vi "GetGlobalDefaultConfiguration_old.vi"(3 "Read defaults?":bool) -> ()   [LabVIEW 2013]
uses:
  QC_MeasurementSetup.vi
panel:
  out "Configuration File Striptest":path
  out "Configuration File Cis":path
  out "Configuration File Stability":path
  out "Configuration File CV":path
  out "Configuration File IV":path
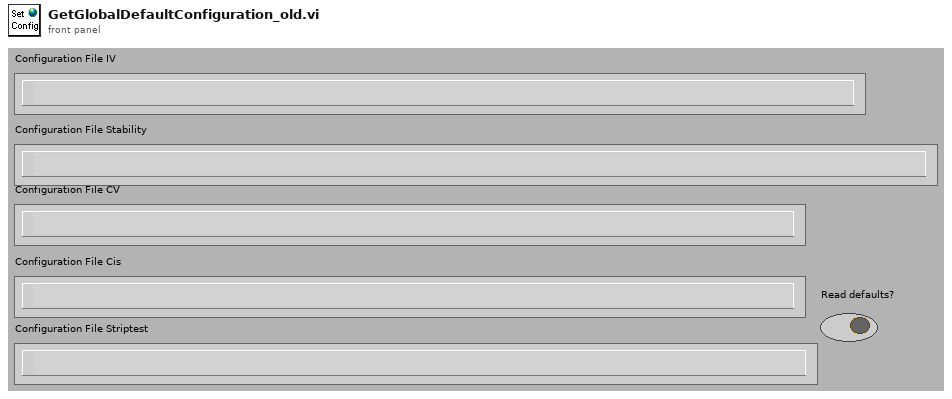
[diagram p1: front panel]
types:
  T1 = cluster{"Supply":refnum<class "SupplyControl.lvclass">, "Arduino":refnum<class "ArduinoControl.lvclass">, "Measurement switch":refnum<class "Switching.lvclass">, "Initial Voltage [V]":dbl, "Final Voltage [V]":dbl, "Step Size [V]":dbl, "Step Interval [s]":i32, "Number Of Steps":u32, "Ramp down steps [V]":dbl, "Ramp down Interval [s]":i32, "hold steps":i32, "Set Current Limit?":bool, "Current Limit [µA]":dbl, "Temperature Readout":enum16{"Read Arduino", "Enter manually"}, "Supply Name":string, "V_breakdown Limit [V]":dbl, "Measurement switch used?":bool}
  T2 = cluster{"Supply":refnum<class "SupplyControl.lvclass">, "LCR":refnum<class "LCRControl.lvclass">, "Arduino":refnum<class "ArduinoControl.lvclass">, "Measurement switch":refnum<class "Switching.lvclass">, "Initial Voltage [V]":dbl, "Final Voltage [V]":dbl, "Step Size [V]":dbl, "Step Interval [s]":i32, "Number Of Steps":u32, "AC frequency [Hz]":i32, "RC Configuration":u16, "AC amplitude [V]":dbl, "Ramp down steps [V]":dbl, "Ramp down Interval [s]":i32, "Set Current Limit?":bool, "Current Limit [µA]":dbl, "Temperature Readout":enum16{"Read Arduino", "Enter manually"}, "Supply Name":string, "LCR Name":string, "V_depletion Limit [V]":dbl, "Measurement switch used?":bool}
  T3 = cluster{"Supply":refnum<class "SupplyControl.lvclass">, "DMM":refnum<class "MultimeterControl.lvclass">, "DUT switch":refnum<class "Switching.lvclass">, "Arduino":refnum<class "ArduinoControl.lvclass">, "Measurement switch":refnum<class "Switching.lvclass">, "Voltage [V]":dbl, "Measurement Interval [s]":i32, "Test Duration":u32, "Ramp up steps [V]":dbl, "Ramp up Interval [s]":u32, "Ramp down steps [V]":dbl, "Ramp down Interval [s]":i32, "Set Current Limit?":bool, "Current Limit [µA]":dbl, "Temperature Readout":enum16{"Read Arduino", "Enter manually"}, "Supply Name":string, "DMM Name":string, "Maximum current fluctuation [%]":dbl, "Measurement switch used?":bool, "DUT switch used?":bool}
  T4 = cluster{"Supply":refnum<class "SupplyControl.lvclass">, "LCR":refnum<class "LCRControl.lvclass">, "Arduino":refnum<class "ArduinoControl.lvclass">, "Measurement switch":refnum<class "Switching.lvclass">, "Initial Voltage [V]":dbl, "Final Voltage [V]":dbl, "Step Size [V]":dbl, "Step Interval [s]":i32, "Number Of Steps":u32, "AC frequency [Hz]":i32, "RC Configuration":u16, "AC amplitude [V]":dbl, "Ramp down steps [V]":dbl, "Ramp down Interval [s]":i32, "Set Current Limit?":bool, "Current Limit [µA]":dbl, "Temperature Readout":enum16{"Read Arduino", "Enter manually"}, "Supply Name":string, "LCR Name":string, "C_is Limit [pF/cm]":dbl, "Measurement switch used?":bool}
  T5 = cluster{"Bias Supply":refnum<class "SupplyControl.lvclass">, "SMU":refnum<class "SupplyControl.lvclass">, "LCR":refnum<class "LCRControl.lvclass">, "ProbeStation":refnum<class "ProbeStationControl.lvclass">, "Arduino":refnum<class "ArduinoControl.lvclass">, "Measurement switch":refnum<class "Switching.lvclass">, "Probe Card Channels":i32, "Bias Voltage [V]":dbl, "First strip":i32, "Last strip":i32, "Base Voltage [V]":dbl, "Base Ramp Step [V]":dbl, "Base Ramp Interval [ms]":u32, "High Voltage [V]":dbl, "High Ramp Step [V]":dbl, "High Ramp Interval [ms]":u32, "AC frequency [Hz]":i32, "AC amplitude [V]":dbl, "RC Configuration":u16, "Single Needle":bool, "Temperature Readout":enum16{"Read Arduino", "Enter manually"}, "Fraction of good strips [%]":dbl, "Measurement switch used?":bool, "Matrix X Channels":cluster{"Mux1 C1":i32, "Mux1 C2":i32, "Mux2 C1":i32, "Mux2 C2":i32}, "Pinholes Y/N":bool, "Capacitance Y/N":bool, "Resistance Y/N":bool, "Bias Supply Name":string, "SMU Name":string, "LCR Name":string}
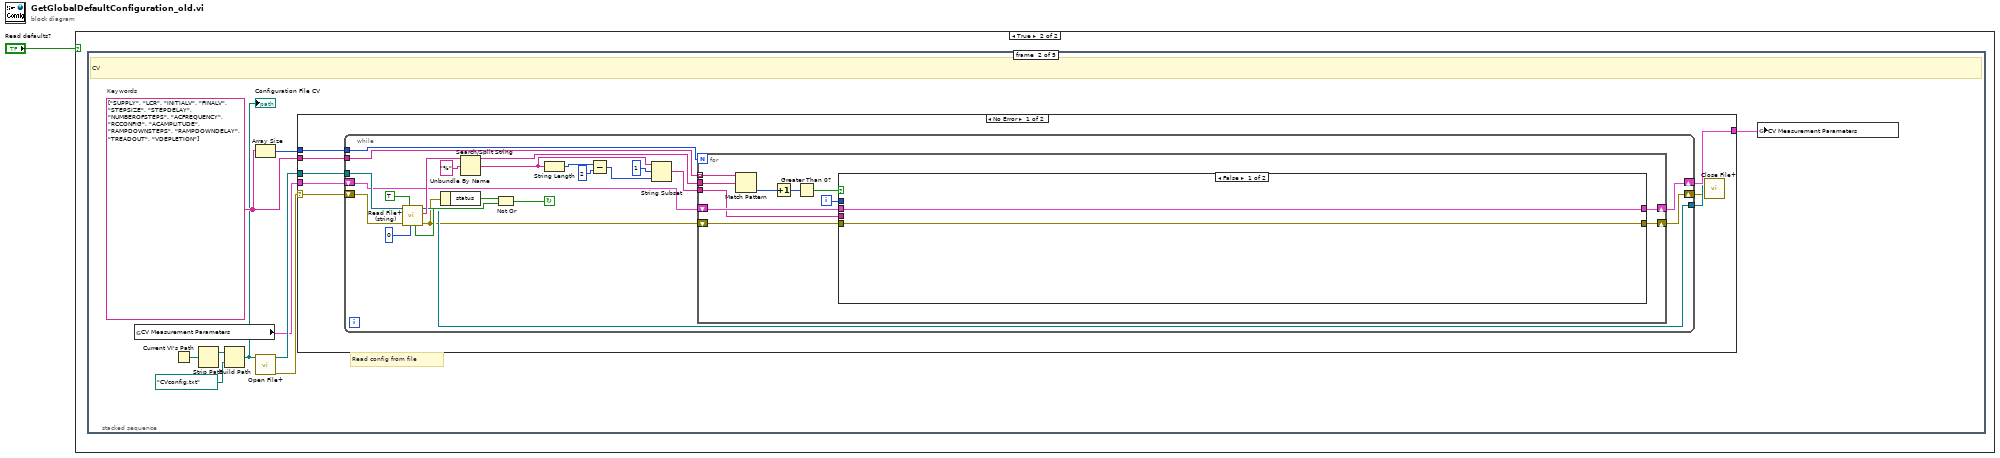
[diagram p0: block diagram]
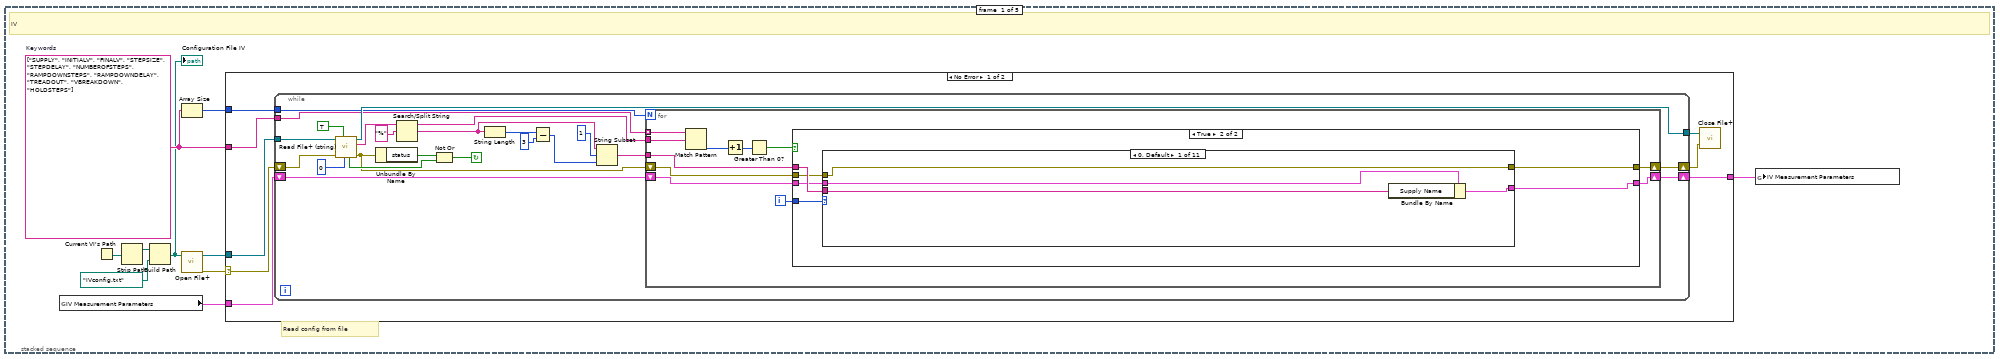
[diagram p3: hidden frame]
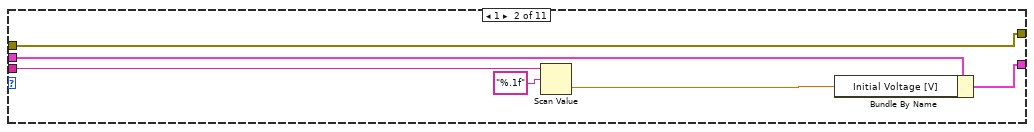
[diagram p5: hidden frame]
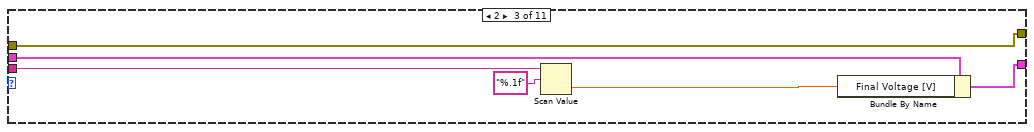
[diagram p6: hidden frame]
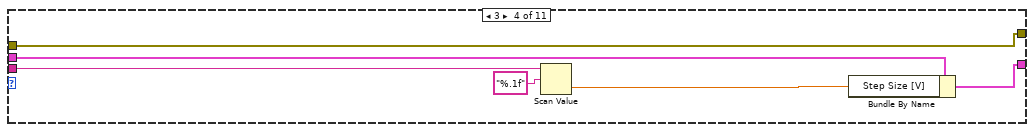
[diagram p7: hidden frame]
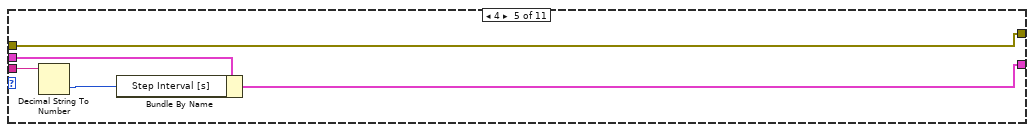
[diagram p8: hidden frame]
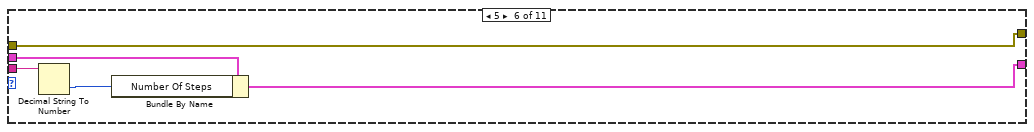
[diagram p9: hidden frame]
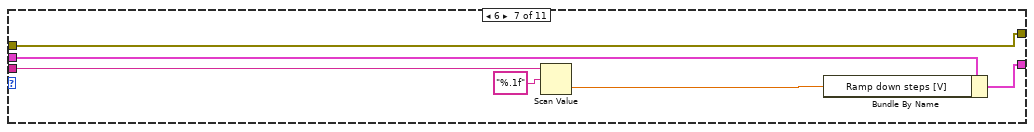
[diagram p10: hidden frame]
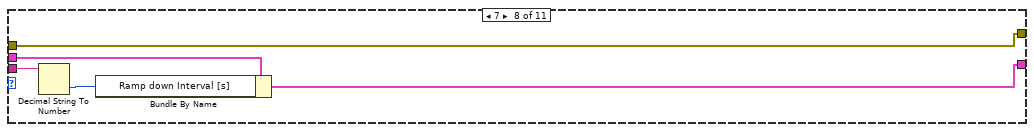
[diagram p11: hidden frame]
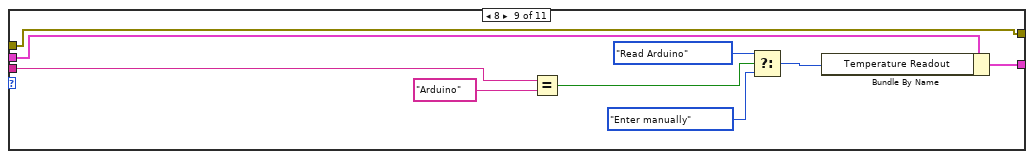
[diagram p12: hidden frame]
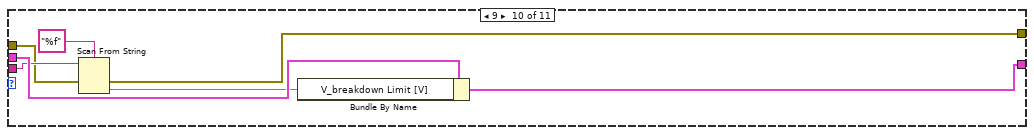
[diagram p13: hidden frame]
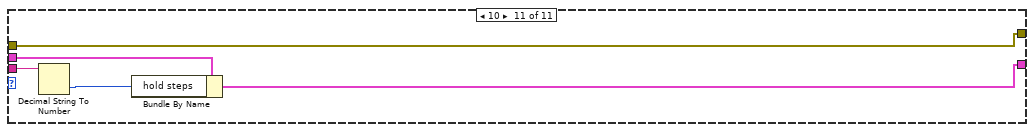
[diagram p14: hidden frame]
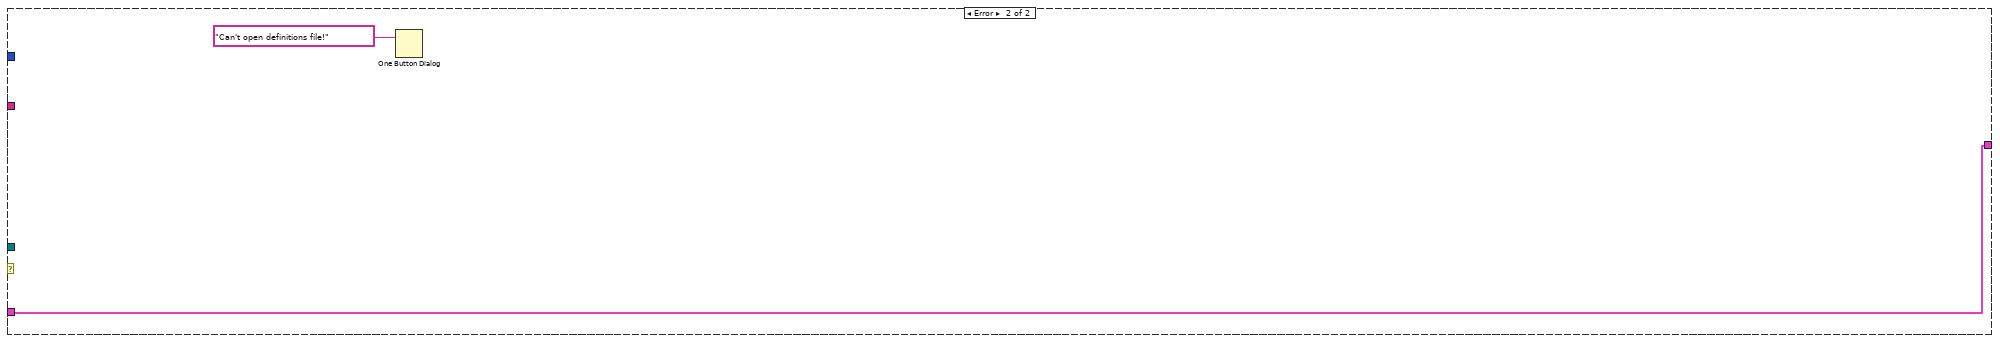
[diagram p15: hidden frame]
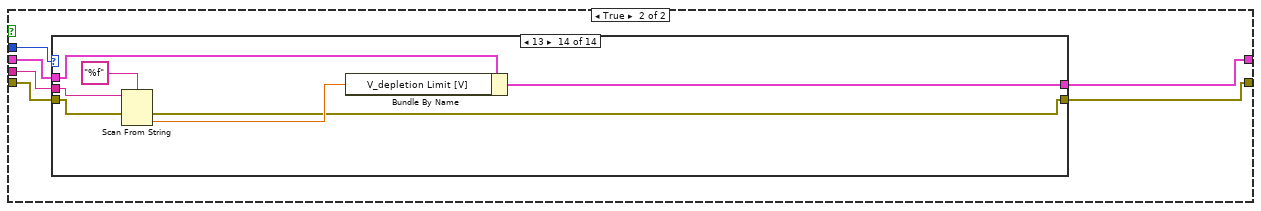
[diagram p16: hidden frame]
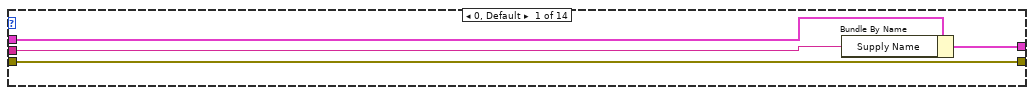
[diagram p17: hidden frame]
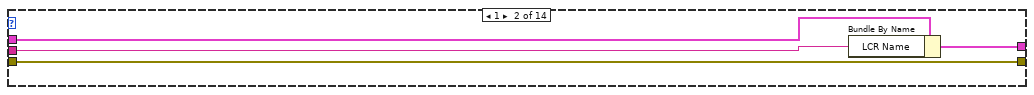
[diagram p18: hidden frame]
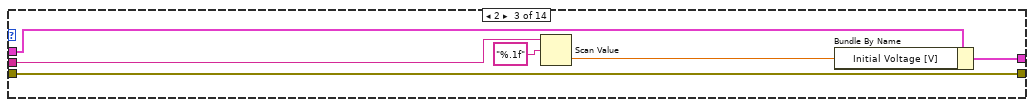
[diagram p19: hidden frame]
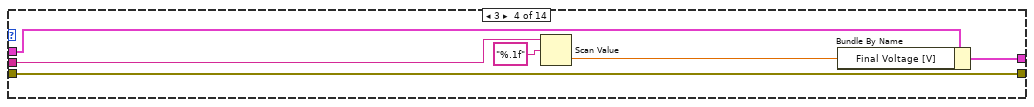
[diagram p20: hidden frame]
diagram:
  n1 = case shown="True" "Read defaults?" {
    frame False {
    }
    frame True {
      n2 = stacked-sequence {
        frame #0 {
          w11 = string[] ["SUPPLY", "INITIALV", "FINALV", "STEPSIZE", "STEPDELAY", "NUMBEROFSTEPS", "RAMPDOWNSTEPS", "RAMPDOWNDELAY", "TREADOUT", "VBREAKDOWN", "HOLDSTEPS"]  # Keywords
          # "Read config from file"
          # "IV"
          n3 = global read "QC_MeasurementSetup.vi" "IV Measurement Parameters"() -> (w2:T1)
          n4 = Current VI's Path() -> (path=w6:path)
          n5 = Strip Path(path=w6) -> (stripped path=w5:path)  [unwired: 1 out]
          n6 = Build Path(base path=w5, name or relative path=path "IVconfig.txt") -> (appended path=w4:path)
          "Configuration File IV" <- w4
          n7 = Array Size(array=w11) -> (size(s)=w10:i32)
          n8 = call <vilib>:"Open File+.vi"("file path (\" \")"=w4) -> ("error out"=w7:errorcluster, "refnum"=w8:refnum<file>)  [unwired: 7 in, 2 out]
          n9 = case shown="No Error" w7 {
            selector: w7 -> [w12 _]
            tunnel: w8 -> [w19 _]
            tunnel: w11 -> [w18 _]
            tunnel: w10 -> [w17 _]
            tunnel: w2 -> [w16 w126]
            tunnel: [w15 w126] -> w3
            frame No Error {
              n10 = while {
                shift-left: w16 -> [w25]
                shift-right: [w23] -> w15
                tunnel: w17 -> [w22]
                tunnel: w18 -> [w28]
                tunnel: [w33] -> w14
                tunnel: w19 -> [w39]
                shift-right: [w20] -> w13
                shift-left: w12 -> [w32]
                stop <- w35 continue-if-true
                n11 = call <vilib>:"Read File+ (string).vi"("count"=0, "line mode (characters:F)"=TRUE, "error in (no error)"=w32, "refnum"=w39) -> ("error out"=w21:errorcluster, "string"=w34:string, "dup refnum"=w33:refnum<file>, "EOF?"=w37:bool)  [unwired: 3 in, 1 out]
                n12 = Unbundle By Name(w21) -> ("status"=w36:bool)
                n13 = Search/Split String(string=w34, search string/char (-)="%" ("search char (-)")) -> (substring before match=w27:string, match + rest of string=w40:string)  [unwired: 1 in, 1 out]
                n14 = Not Or(1:w37, 2:w36) -> (0:w35:bool)
                n15 = String Length(string=w40) -> (length=w26:i32)
                n16 = Subtract(x=w26, y=3) -> (x-y=w29:i32)
                n17 = String Subset(string=w40, offset (0)=1, length (rest)=w29) -> (substring=w24:string)
                n18 = for {
                  N: w22 -> [_]
                  tunnel: w28 -> [w51] mode=indexing
                  tunnel: w27 -> [w46]
                  shift-right: [w47] -> w23
                  shift-left: w25 -> [w48]
                  tunnel: w24 -> [w45]
                  shift-right: [w43] -> w20
                  shift-left: w21 -> [w44]
                  i -> [w49]
                  n19 = Match Pattern(string=w51, regular expression=w46) -> (offset past match=w52:i32)  [unwired: 1 in, 3 out]
                  n20 = Increment(x=w52) -> (x+1=w53:i32)
                  n21 = Greater Than 0?(x=w53) -> (x > 0?=w50:bool)
                  n22 = case shown="True" w50 {
                    tunnel: w49 -> [_ w61]
                    tunnel: w45 -> [_ w60]
                    tunnel: w48 -> [w55 w59]
                    tunnel: [w55 w58] -> w47
                    tunnel: w44 -> [w54 w57]
                    tunnel: [w54 w56] -> w43
                    frame False {
                    }
                    frame True {
                      n23 = case shown="0, Default" w61 {
                        tunnel: w60 -> [w63 w69 w74 w80 w86 w91 w96 w102 w111 w118 w122]
                        tunnel: w59 -> [w64 w71 w77 w83 w88 w93 w99 w104 w113 w120 w125]
                        tunnel: [w65 w70 w76 w82 w87 w92 w98 w103 w112 w119 w124] -> w58
                        tunnel: w57 -> [w62 w66 w72 w78 w84 w89 w94 w100 w110 w115 w121]
                        tunnel: [w62 w66 w72 w78 w84 w89 w94 w100 w110 w114 w121] -> w56
                        frame 0, Default {
                          n24 = Bundle By Name(cluster=w64, "Supply Name"=w63) -> (w65:T1)
                        }
                        frame 1 {
                          n25 = Scan Value(string=w69, format string="%.1f") -> (value=w68:dbl)  [unwired: 1 in, 1 out]
                          n26 = Bundle By Name(cluster=w71, "Initial Voltage [V]"=w68) -> (w70:T1)
                        }
                        frame 2 {
                          n27 = Scan Value(string=w74, format string="%.1f") -> (value=w73:dbl)  [unwired: 1 in, 1 out]
                          n28 = Bundle By Name(cluster=w77, "Final Voltage [V]"=w73) -> (w76:T1)
                        }
                        frame 3 {
                          n29 = Scan Value(string=w80, format string="%.1f") -> (value=w79:dbl)  [unwired: 1 in, 1 out]
                          n30 = Bundle By Name(cluster=w83, "Step Size [V]"=w79) -> (w82:T1)
                        }
                        frame 4 {
                          n31 = Decimal String To Number(string=w86) -> (number=w85:i32)  [unwired: 2 in, 1 out]
                          n32 = Bundle By Name(cluster=w88, "Step Interval [s]"=w85) -> (w87:T1)
                        }
                        frame 5 {
                          n33 = Decimal String To Number(string=w91) -> (number=w90:i32)  [unwired: 2 in, 1 out]
                          n34 = Bundle By Name(cluster=w93, "Number Of Steps"=w90) -> (w92:T1)
                        }
                        frame 6 {
                          n35 = Scan Value(string=w96, format string="%.1f") -> (value=w95:dbl)  [unwired: 1 in, 1 out]
                          n36 = Bundle By Name(cluster=w99, "Ramp down steps [V]"=w95) -> (w98:T1)
                        }
                        frame 7 {
                          n37 = Decimal String To Number(string=w102) -> (number=w101:i32)  [unwired: 2 in, 1 out]
                          n38 = Bundle By Name(cluster=w104, "Ramp down Interval [s]"=w101) -> (w103:T1)
                        }
                        frame 8 {
                          n39 = Equal?(x=w111, y="Arduino") -> (x = y?=w108:bool)
                          n40 = Select(t=enum16{"Read Arduino", "Enter manually"}."Read Arduino" ("Temperature Readout"), s=w108, f=enum16{"Read Arduino", "Enter manually"}."Enter manually" ("Temperature Readout")) -> (s? t:f=w105:enum16{"Read Arduino", "Enter manually"})
                          n41 = Bundle By Name(cluster=w113, "Temperature Readout"=w105) -> (w112:T1)
                        }
                        frame 9 {
                          n42 = Scan From String(format string="%f", input string=w118, error in=w115) -> (error out=w114:errorcluster, output 1=w117:dbl)  [unwired: 2 in, 2 out]
                          n43 = Bundle By Name(cluster=w120, "V_breakdown Limit [V]"=w117) -> (w119:T1)
                        }
                        frame 10 {
                          n44 = Decimal String To Number(string=w122) -> (number=w123:i32)  [unwired: 2 in, 1 out]
                          n45 = Bundle By Name(cluster=w125, "hold steps"=w123) -> (w124:T1)
                        }
                      }
                    }
                  }
                }
              }
              n46 = call <vilib>:"Close File+.vi"("error in (no error)"=w13, "refnum"=w14) -> ()  [unwired: 3 in, 3 out]
            }
            frame Error {
              n47 = One Button Dialog(message="Can't open definitions file!") -> ()  [unwired: 1 in, 1 out]
            }
          }
          n48 = global write "QC_MeasurementSetup.vi" "IV Measurement Parameters"(w3) -> ()
        }
        frame #1 {
          w137 = string[] ["SUPPLY", "LCR", "INITIALV", "FINALV", "STEPSIZE", "STEPDELAY", "NUMBEROFSTEPS", "ACFREQUENCY", "RCCONFIG", "ACAMPLITUDE", "RAMPDOWNSTEPS", "RAMPDOWNDELAY", "TREADOUT", "VDEPLETION"]  # Keywords
          # "Read config from file"
          # "CV"
          n49 = global read "QC_MeasurementSetup.vi" "CV Measurement Parameters"() -> (w128:T2)
          n50 = Current VI's Path() -> (path=w132:path)
          n51 = Strip Path(path=w132) -> (stripped path=w131:path)  [unwired: 1 out]
          n52 = Build Path(base path=w131, name or relative path=path "CVconfig.txt") -> (appended path=w130:path)
          "Configuration File CV" <- w130
          n53 = Array Size(array=w137) -> (size(s)=w136:i32)
          n54 = call <vilib>:"Open File+.vi"("file path (\" \")"=w130) -> ("error out"=w133:errorcluster, "refnum"=w134:refnum<file>)  [unwired: 7 in, 2 out]
          n55 = case shown="No Error" w133 {
            selector: w133 -> [w138 _]
            tunnel: w134 -> [w145 _]
            tunnel: w137 -> [w144 _]
            tunnel: w136 -> [w143 _]
            tunnel: w128 -> [w142 w271]
            tunnel: [w141 w271] -> w129
            frame No Error {
              n56 = while {
                shift-left: w142 -> [w151]
                shift-right: [w149] -> w141
                tunnel: w143 -> [w148]
                tunnel: w144 -> [w154]
                tunnel: [w159] -> w140
                tunnel: w145 -> [w165]
                shift-right: [w146] -> w139
                shift-left: w138 -> [w158]
                stop <- w161 continue-if-true
                n57 = call <vilib>:"Read File+ (string).vi"("count"=0, "line mode (characters:F)"=TRUE, "error in (no error)"=w158, "refnum"=w165) -> ("error out"=w147:errorcluster, "string"=w160:string, "dup refnum"=w159:refnum<file>, "EOF?"=w163:bool)  [unwired: 3 in, 1 out]
                n58 = Unbundle By Name(w147) -> ("status"=w162:bool)
                n59 = Search/Split String(string=w160, search string/char (-)="%" ("search char (-)")) -> (substring before match=w153:string, match + rest of string=w166:string)  [unwired: 1 in, 1 out]
                n60 = Not Or(1:w163, 2:w162) -> (0:w161:bool)
                n61 = String Length(string=w166) -> (length=w152:i32)
                n62 = Subtract(x=w152, y=2) -> (x-y=w155:i32)
                n63 = String Subset(string=w166, offset (0)=1, length (rest)=w155) -> (substring=w150:string)
                n64 = for {
                  N: w148 -> [_]
                  tunnel: w154 -> [w177] mode=indexing
                  tunnel: w153 -> [w172]
                  shift-right: [w173] -> w149
                  shift-left: w151 -> [w174]
                  tunnel: w150 -> [w171]
                  shift-right: [w169] -> w146
                  shift-left: w147 -> [w170]
                  i -> [w175]
                  n65 = Match Pattern(string=w177, regular expression=w172) -> (offset past match=w178:i32)  [unwired: 1 in, 3 out]
                  n66 = Increment(x=w178) -> (x+1=w179:i32)
                  n67 = Greater Than 0?(x=w179) -> (x > 0?=w176:bool)
                  n68 = case shown="False" w176 {
                    tunnel: w175 -> [_ w187]
                    tunnel: w171 -> [_ w186]
                    tunnel: w174 -> [w181 w185]
                    tunnel: [w181 w184] -> w173
                    tunnel: w170 -> [w180 w183]
                    tunnel: [w180 w182] -> w169
                    frame False {
                    }
                    frame True {
                      n69 = case shown="13" w187 {
                        tunnel: w186 -> [w189 w193 w199 w204 w210 w216 w221 w226 w234 w243 w246 w252 w261 w268]
                        tunnel: w185 -> [w190 w194 w201 w207 w213 w218 w223 w228 w237 w241 w249 w254 w263 w264]
                        tunnel: [w191 w195 w200 w206 w212 w217 w222 w227 w236 w239 w248 w253 w262 w265] -> w184
                        tunnel: w183 -> [w188 w192 w196 w202 w208 w214 w219 w224 w229 w238 w244 w250 w260 w267]
                        tunnel: [w188 w192 w196 w202 w208 w214 w219 w224 w229 w238 w244 w250 w260 w266] -> w182
                        frame 0, Default {
                          n70 = Bundle By Name(cluster=w190, "Supply Name"=w189) -> (w191:T2)
                        }
                        frame 1 {
                          n71 = Bundle By Name(cluster=w194, "LCR Name"=w193) -> (w195:T2)
                        }
                        frame 2 {
                          n72 = Scan Value(string=w199, format string="%.1f") -> (value=w198:dbl)  [unwired: 1 in, 1 out]
                          n73 = Bundle By Name(cluster=w201, "Initial Voltage [V]"=w198) -> (w200:T2)
                        }
                        frame 3 {
                          n74 = Scan Value(string=w204, format string="%.1f") -> (value=w203:dbl)  [unwired: 1 in, 1 out]
                          n75 = Bundle By Name(cluster=w207, "Final Voltage [V]"=w203) -> (w206:T2)
                        }
                        frame 4 {
                          n76 = Scan Value(string=w210, format string="%.1f") -> (value=w209:dbl)  [unwired: 1 in, 1 out]
                          n77 = Bundle By Name(cluster=w213, "Step Size [V]"=w209) -> (w212:T2)
                        }
                        frame 5 {
                          n78 = Decimal String To Number(string=w216) -> (number=w215:i32)  [unwired: 2 in, 1 out]
                          n79 = Bundle By Name(cluster=w218, "Step Interval [s]"=w215) -> (w217:T2)
                        }
                        frame 6 {
                          n80 = Decimal String To Number(string=w221) -> (number=w220:i32)  [unwired: 2 in, 1 out]
                          n81 = Bundle By Name(cluster=w223, "Number Of Steps"=w220) -> (w222:T2)
                        }
                        frame 7 {
                          n82 = Decimal String To Number(string=w226) -> (number=w225:i32)  [unwired: 2 in, 1 out]
                          n83 = Bundle By Name(cluster=w228, "AC frequency [Hz]"=w225) -> (w227:T2)
                        }
                        frame 8 {
                          w233 = u16 0 items=["serial", "parallel"] ("RC Configuration")
                          w232 = u16 1 items=["serial", "parallel"] ("RC Configuration")
                          n84 = Equal?(x=w234, y="serial") -> (x = y?=w231:bool)
                          n85 = Select(t=w233, s=w231, f=w232) -> (s? t:f=w230:u16)
                          n86 = Bundle By Name(cluster=w237, "RC Configuration"=w230) -> (w236:T2)
                        }
                        frame 9 {
                          n87 = Scan Value(string=w243, format string="%.1f") -> (value=w240:dbl)  [unwired: 1 in, 1 out]
                          n88 = Bundle By Name(cluster=w241, "AC amplitude [V]"=w240) -> (w239:T2)
                        }
                        frame 10 {
                          n89 = Scan Value(string=w246, format string="%.1f") -> (value=w245:dbl)  [unwired: 1 in, 1 out]
                          n90 = Bundle By Name(cluster=w249, "Ramp down steps [V]"=w245) -> (w248:T2)
                        }
                        frame 11 {
                          n91 = Decimal String To Number(string=w252) -> (number=w251:i32)  [unwired: 2 in, 1 out]
                          n92 = Bundle By Name(cluster=w254, "Ramp down Interval [s]"=w251) -> (w253:T2)
                        }
                        frame 12 {
                          n93 = Equal?(x=w261, y="Arduino") -> (x = y?=w258:bool)
                          n94 = Select(t=enum16{"Read Arduino", "Enter manually"}."Read Arduino" ("Temperature Readout"), s=w258, f=enum16{"Read Arduino", "Enter manually"}."Enter manually" ("Temperature Readout")) -> (s? t:f=w255:enum16{"Read Arduino", "Enter manually"})
                          n95 = Bundle By Name(cluster=w263, "Temperature Readout"=w255) -> (w262:T2)
                        }
                        frame 13 {
                          n96 = Scan From String(format string="%f", input string=w268, error in=w267) -> (error out=w266:errorcluster, output 1=w270:dbl)  [unwired: 2 in, 2 out]
                          n97 = Bundle By Name(cluster=w264, "V_depletion Limit [V]"=w270) -> (w265:T2)
                        }
                      }
                    }
                  }
                }
              }
              n98 = call <vilib>:"Close File+.vi"("error in (no error)"=w139, "refnum"=w140) -> ()  [unwired: 3 in, 3 out]
            }
            frame Error {
              n99 = One Button Dialog(message="Can't open definitions file!") -> ()  [unwired: 1 in, 1 out]
            }
          }
          n100 = global write "QC_MeasurementSetup.vi" "CV Measurement Parameters"(w129) -> ()
        }
        frame #2 {
          w282 = string[] ["SUPPLY", "VOLTAGE", "INTERVAL", "DURATION", "RAMPUPSTEPS", "RAMPUPDELAY", "RAMPDOWNSTEPS", "RAMPDOWNDELAY", "TREADOUT", "IFLUCTUATIONS"]  # Keywords
          # "Read config from file"
          # "STABILITY"
          n101 = global read "QC_MeasurementSetup.vi" "Current Stability Measurement Parameters"() -> (w273:T3)
          n102 = Current VI's Path() -> (path=w277:path)
          n103 = Strip Path(path=w277) -> (stripped path=w276:path)  [unwired: 1 out]
          n104 = Build Path(base path=w276, name or relative path=path "STABILITYconfig.txt") -> (appended path=w275:path)
          "Configuration File Stability" <- w275
          n105 = Array Size(array=w282) -> (size(s)=w281:i32)
          n106 = call <vilib>:"Open File+.vi"("file path (\" \")"=w275) -> ("error out"=w278:errorcluster, "refnum"=w279:refnum<file>)  [unwired: 7 in, 2 out]
          n107 = case shown="No Error" w278 {
            selector: w278 -> [w283 _]
            tunnel: w279 -> [w290 _]
            tunnel: w282 -> [w289 _]
            tunnel: w281 -> [w288 _]
            tunnel: w273 -> [w287 w391]
            tunnel: [w286 w391] -> w274
            frame No Error {
              n108 = while {
                shift-left: w287 -> [w296]
                shift-right: [w294] -> w286
                tunnel: w288 -> [w293]
                tunnel: w289 -> [w299]
                tunnel: [w304] -> w285
                tunnel: w290 -> [w310]
                shift-right: [w291] -> w284
                shift-left: w283 -> [w303]
                stop <- w306 continue-if-true
                n109 = call <vilib>:"Read File+ (string).vi"("count"=0, "line mode (characters:F)"=TRUE, "error in (no error)"=w303, "refnum"=w310) -> ("error out"=w292:errorcluster, "string"=w305:string, "dup refnum"=w304:refnum<file>, "EOF?"=w308:bool)  [unwired: 3 in, 1 out]
                n110 = Unbundle By Name(w292) -> ("status"=w307:bool)
                n111 = Search/Split String(string=w305, search string/char (-)="%" ("search char (-)")) -> (substring before match=w298:string, match + rest of string=w311:string)  [unwired: 1 in, 1 out]
                n112 = Not Or(1:w308, 2:w307) -> (0:w306:bool)
                n113 = String Length(string=w311) -> (length=w297:i32)
                n114 = Subtract(x=w297, y=3) -> (x-y=w300:i32)
                n115 = String Subset(string=w311, offset (0)=1, length (rest)=w300) -> (substring=w295:string)
                n116 = for {
                  N: w293 -> [_]
                  tunnel: w299 -> [w322] mode=indexing
                  tunnel: w298 -> [w317]
                  shift-right: [w318] -> w294
                  shift-left: w296 -> [w319]
                  tunnel: w295 -> [w316]
                  shift-right: [w314] -> w291
                  shift-left: w292 -> [w315]
                  i -> [w320]
                  n117 = Match Pattern(string=w322, regular expression=w317) -> (offset past match=w323:i32)  [unwired: 1 in, 3 out]
                  n118 = Increment(x=w323) -> (x+1=w324:i32)
                  n119 = Greater Than 0?(x=w324) -> (x > 0?=w321:bool)
                  n120 = case shown="True" w321 {
                    tunnel: w320 -> [_ w332]
                    tunnel: w316 -> [_ w331]
                    tunnel: w319 -> [w326 w330]
                    tunnel: [w326 w329] -> w318
                    tunnel: w315 -> [w325 w328]
                    tunnel: [w325 w327] -> w314
                    frame False {
                    }
                    frame True {
                      n121 = case shown="7" w332 {
                        tunnel: w331 -> [w333 w340 w344 w349 w355 w361 w366 w372 w381 w387]
                        tunnel: w330 -> [w335 w342 w347 w352 w358 w363 w369 w374 w383 w388]
                        tunnel: [w336 w341 w346 w351 w357 w362 w368 w373 w382 w386] -> w329
                        tunnel: w328 -> [w334 w337 w345 w350 w356 w359 w364 w370 w380 w384]
                        tunnel: [w334 w337 w345 w350 w356 w359 w364 w370 w380 w385] -> w327
                        frame 0, Default {
                          n122 = Bundle By Name(cluster=w335, "Supply Name"=w333) -> (w336:T3)
                        }
                        frame 1 {
                          n123 = Scan Value(string=w340, format string="%.1f") -> (value=w339:dbl)  [unwired: 1 in, 1 out]
                          n124 = Bundle By Name(cluster=w342, "Voltage [V]"=w339) -> (w341:T3)
                        }
                        frame 2 {
                          n125 = Decimal String To Number(string=w344) -> (number=w343:i32)  [unwired: 2 in, 1 out]
                          n126 = Bundle By Name(cluster=w347, "Measurement Interval [s]"=w343) -> (w346:T3)
                        }
                        frame 3 {
                          n127 = Decimal String To Number(string=w349) -> (number=w348:i32)  [unwired: 2 in, 1 out]
                          n128 = Bundle By Name(cluster=w352, "Test Duration"=w348) -> (w351:T3)
                        }
                        frame 4 {
                          n129 = Scan Value(string=w355, format string="%.1f") -> (value=w353:dbl)  [unwired: 1 in, 1 out]
                          n130 = Bundle By Name(cluster=w358, "Ramp up steps [V]"=w353) -> (w357:T3)
                        }
                        frame 5 {
                          n131 = Decimal String To Number(string=w361) -> (number=w360:i32)  [unwired: 2 in, 1 out]
                          n132 = Bundle By Name(cluster=w363, "Ramp up Interval [s]"=w360) -> (w362:T3)
                        }
                        frame 6 {
                          n133 = Scan Value(string=w366, format string="%.1f") -> (value=w365:dbl)  [unwired: 1 in, 1 out]
                          n134 = Bundle By Name(cluster=w369, "Ramp down steps [V]"=w365) -> (w368:T3)
                        }
                        frame 7 {
                          n135 = Decimal String To Number(string=w372) -> (number=w371:i32)  [unwired: 2 in, 1 out]
                          n136 = Bundle By Name(cluster=w374, "Ramp down Interval [s]"=w371) -> (w373:T3)
                        }
                        frame 8 {
                          n137 = Equal?(x=w381, y="Arduino") -> (x = y?=w378:bool)
                          n138 = Select(t=enum16{"Read Arduino", "Enter manually"}."Read Arduino" ("Temperature Readout"), s=w378, f=enum16{"Read Arduino", "Enter manually"}."Enter manually" ("Temperature Readout")) -> (s? t:f=w375:enum16{"Read Arduino", "Enter manually"})
                          n139 = Bundle By Name(cluster=w383, "Temperature Readout"=w375) -> (w382:T3)
                        }
                        frame 9 {
                          n140 = Scan From String(format string="%f", input string=w387, error in=w384) -> (error out=w385:errorcluster, output 1=w390:dbl)  [unwired: 2 in, 2 out]
                          n141 = Bundle By Name(cluster=w388, "Maximum current fluctuation [%]"=w390) -> (w386:T3)
                        }
                      }
                    }
                  }
                }
              }
              n142 = call <vilib>:"Close File+.vi"("error in (no error)"=w284, "refnum"=w285) -> ()  [unwired: 3 in, 3 out]
            }
            frame Error {
              n143 = One Button Dialog(message="Can't open definitions file!") -> ()  [unwired: 1 in, 1 out]
            }
          }
          n144 = global write "QC_MeasurementSetup.vi" "Current Stability Measurement Parameters"(w274) -> ()
        }
        frame #3 {
          w402 = string[] ["SUPPLY", "LCR", "INITIALV", "FINALV", "STEPSIZE", "STEPDELAY", "NUMBEROFSTEPS", "ACFREQUENCY", "RCCONFIG", "ACAMPLITUDE", "RAMPDOWNSTEPS", "RAMPDOWNDELAY", "TREADOUT", "CISLIMIT"]  # Keywords
          # "Read config from file"
          # "CIS"
          n145 = global read "QC_MeasurementSetup.vi" "Cis Measurement Parameters"() -> (w393:T4)
          n146 = Current VI's Path() -> (path=w397:path)
          n147 = Strip Path(path=w397) -> (stripped path=w396:path)  [unwired: 1 out]
          n148 = Build Path(base path=w396, name or relative path=path "CISconfig.txt") -> (appended path=w395:path)
          "Configuration File Cis" <- w395
          n149 = Array Size(array=w402) -> (size(s)=w401:i32)
          n150 = call <vilib>:"Open File+.vi"("file path (\" \")"=w395) -> ("error out"=w398:errorcluster, "refnum"=w399:refnum<file>)  [unwired: 7 in, 2 out]
          n151 = case shown="No Error" w398 {
            selector: w398 -> [w403 _]
            tunnel: w399 -> [w410 _]
            tunnel: w402 -> [w409 _]
            tunnel: w401 -> [w408 _]
            tunnel: w393 -> [w407 w536]
            tunnel: [w406 w536] -> w394
            frame No Error {
              n152 = while {
                shift-left: w407 -> [w416]
                shift-right: [w414] -> w406
                tunnel: w408 -> [w413]
                tunnel: w409 -> [w419]
                tunnel: [w424] -> w405
                tunnel: w410 -> [w430]
                shift-right: [w411] -> w404
                shift-left: w403 -> [w423]
                stop <- w426 continue-if-true
                n153 = call <vilib>:"Read File+ (string).vi"("count"=0, "line mode (characters:F)"=TRUE, "error in (no error)"=w423, "refnum"=w430) -> ("error out"=w412:errorcluster, "string"=w425:string, "dup refnum"=w424:refnum<file>, "EOF?"=w428:bool)  [unwired: 3 in, 1 out]
                n154 = Unbundle By Name(w412) -> ("status"=w427:bool)
                n155 = Search/Split String(string=w425, search string/char (-)="%" ("search char (-)")) -> (substring before match=w418:string, match + rest of string=w431:string)  [unwired: 1 in, 1 out]
                n156 = Not Or(1:w428, 2:w427) -> (0:w426:bool)
                n157 = String Length(string=w431) -> (length=w417:i32)
                n158 = Subtract(x=w417, y=3) -> (x-y=w420:i32)
                n159 = String Subset(string=w431, offset (0)=1, length (rest)=w420) -> (substring=w415:string)
                n160 = for {
                  N: w413 -> [_]
                  tunnel: w419 -> [w442] mode=indexing
                  tunnel: w418 -> [w437]
                  shift-right: [w438] -> w414
                  shift-left: w416 -> [w439]
                  tunnel: w415 -> [w436]
                  shift-right: [w434] -> w411
                  shift-left: w412 -> [w435]
                  i -> [w440]
                  n161 = Match Pattern(string=w442, regular expression=w437) -> (offset past match=w443:i32)  [unwired: 1 in, 3 out]
                  n162 = Increment(x=w443) -> (x+1=w444:i32)
                  n163 = Greater Than 0?(x=w444) -> (x > 0?=w441:bool)
                  n164 = case shown="True" w441 {
                    tunnel: w440 -> [_ w452]
                    tunnel: w436 -> [_ w451]
                    tunnel: w439 -> [w446 w450]
                    tunnel: [w446 w449] -> w438
                    tunnel: w435 -> [w445 w448]
                    tunnel: [w445 w447] -> w434
                    frame False {
                    }
                    frame True {
                      n165 = case shown="0, Default" w452 {
                        tunnel: w451 -> [w453 w457 w464 w469 w475 w481 w486 w491 w499 w508 w511 w517 w526 w533]
                        tunnel: w450 -> [w455 w459 w466 w472 w478 w483 w488 w493 w502 w506 w514 w519 w528 w532]
                        tunnel: [w456 w460 w465 w471 w477 w482 w487 w492 w501 w504 w513 w518 w527 w531] -> w449
                        tunnel: w448 -> [w454 w458 w461 w467 w473 w479 w484 w489 w494 w503 w509 w515 w525 w529]
                        tunnel: [w454 w458 w461 w467 w473 w479 w484 w489 w494 w503 w509 w515 w525 w530] -> w447
                        frame 0, Default {
                          n166 = Bundle By Name(cluster=w455, "Supply Name"=w453) -> (w456:T4)
                        }
                        frame 1 {
                          n167 = Bundle By Name(cluster=w459, "LCR Name"=w457) -> (w460:T4)
                        }
                        frame 2 {
                          n168 = Scan Value(string=w464, format string="%.1f") -> (value=w463:dbl)  [unwired: 1 in, 1 out]
                          n169 = Bundle By Name(cluster=w466, "Initial Voltage [V]"=w463) -> (w465:T4)
                        }
                        frame 3 {
                          n170 = Scan Value(string=w469, format string="%.1f") -> (value=w468:dbl)  [unwired: 1 in, 1 out]
                          n171 = Bundle By Name(cluster=w472, "Final Voltage [V]"=w468) -> (w471:T4)
                        }
                        frame 4 {
                          n172 = Scan Value(string=w475, format string="%.1f") -> (value=w474:dbl)  [unwired: 1 in, 1 out]
                          n173 = Bundle By Name(cluster=w478, "Step Size [V]"=w474) -> (w477:T4)
                        }
                        frame 5 {
                          n174 = Decimal String To Number(string=w481) -> (number=w480:i32)  [unwired: 2 in, 1 out]
                          n175 = Bundle By Name(cluster=w483, "Step Interval [s]"=w480) -> (w482:T4)
                        }
                        frame 6 {
                          n176 = Decimal String To Number(string=w486) -> (number=w485:i32)  [unwired: 2 in, 1 out]
                          n177 = Bundle By Name(cluster=w488, "Number Of Steps"=w485) -> (w487:T4)
                        }
                        frame 7 {
                          n178 = Decimal String To Number(string=w491) -> (number=w490:i32)  [unwired: 2 in, 1 out]
                          n179 = Bundle By Name(cluster=w493, "AC frequency [Hz]"=w490) -> (w492:T4)
                        }
                        frame 8 {
                          w498 = u16 0 items=["serial", "parallel"] ("RC Configuration")
                          w497 = u16 1 items=["serial", "parallel"] ("RC Configuration")
                          n180 = Equal?(x=w499, y="serial") -> (x = y?=w496:bool)
                          n181 = Select(t=w498, s=w496, f=w497) -> (s? t:f=w495:u16)
                          n182 = Bundle By Name(cluster=w502, "RC Configuration"=w495) -> (w501:T4)
                        }
                        frame 9 {
                          n183 = Scan Value(string=w508, format string="%.1f") -> (value=w505:dbl)  [unwired: 1 in, 1 out]
                          n184 = Bundle By Name(cluster=w506, "AC amplitude [V]"=w505) -> (w504:T4)
                        }
                        frame 10 {
                          n185 = Scan Value(string=w511, format string="%.1f") -> (value=w510:dbl)  [unwired: 1 in, 1 out]
                          n186 = Bundle By Name(cluster=w514, "Ramp down steps [V]"=w510) -> (w513:T4)
                        }
                        frame 11 {
                          n187 = Decimal String To Number(string=w517) -> (number=w516:i32)  [unwired: 2 in, 1 out]
                          n188 = Bundle By Name(cluster=w519, "Ramp down Interval [s]"=w516) -> (w518:T4)
                        }
                        frame 12 {
                          n189 = Equal?(x=w526, y="Arduino") -> (x = y?=w523:bool)
                          n190 = Select(t=enum16{"Read Arduino", "Enter manually"}."Read Arduino" ("Temperature Readout"), s=w523, f=enum16{"Read Arduino", "Enter manually"}."Enter manually" ("Temperature Readout")) -> (s? t:f=w520:enum16{"Read Arduino", "Enter manually"})
                          n191 = Bundle By Name(cluster=w528, "Temperature Readout"=w520) -> (w527:T4)
                        }
                        frame 13 {
                          n192 = Scan From String(format string="%f", input string=w533, error in=w529) -> (error out=w530:errorcluster, output 1=w535:dbl)  [unwired: 2 in, 2 out]
                          n193 = Bundle By Name(cluster=w532, "C_is Limit [pF/cm]"=w535) -> (w531:T4)
                        }
                      }
                    }
                  }
                }
              }
              n194 = call <vilib>:"Close File+.vi"("error in (no error)"=w404, "refnum"=w405) -> ()  [unwired: 3 in, 3 out]
            }
            frame Error {
              n195 = One Button Dialog(message="Can't open definitions file!") -> ()  [unwired: 1 in, 1 out]
            }
          }
          n196 = global write "QC_MeasurementSetup.vi" "Cis Measurement Parameters"(w394) -> ()
        }
        frame #4 {
          w547 = string[] ["BIASSUPPLY", "SMU", "LCR", "BIASV", "BASEV", "BASERAMP", "BASEINT", "HIGHV", "HIGHRAMP", "HIGHINT", "ACFREQUENCY", "RCCONFIG", "ACAMPLITUDE", "TREADOUT", "GOODSTRIPS", "CARD"]  # Keywords
          # "Read config from file"
          # "STRIPTEST"
          n197 = global read "QC_MeasurementSetup.vi" "Striptest Measurement Parameters"() -> (w539:T5)
          n198 = Current VI's Path() -> (path=w542:path)
          n199 = Strip Path(path=w542) -> (stripped path=w541:path)  [unwired: 1 out]
          n200 = Build Path(base path=w541, name or relative path=path "STRIPTESTconfig.txt") -> (appended path=w538:path)
          "Configuration File Striptest" <- w538
          n201 = Array Size(array=w547) -> (size(s)=w546:i32)
          n202 = call <vilib>:"Open File+.vi"("file path (\" \")"=w538) -> ("error out"=w543:errorcluster, "refnum"=w544:refnum<file>)  [unwired: 7 in, 2 out]
          n203 = case shown="No Error" w543 {
            selector: w543 -> [w548 _]
            tunnel: w544 -> [w555 _]
            tunnel: w547 -> [w554 _]
            tunnel: w546 -> [w553 _]
            tunnel: w539 -> [w552 w690]
            tunnel: [w551 w690] -> w540
            frame No Error {
              n204 = while {
                shift-left: w552 -> [w561]
                shift-right: [w559] -> w551
                tunnel: w553 -> [w558]
                tunnel: w554 -> [w564]
                tunnel: [w569] -> w550
                tunnel: w555 -> [w575]
                shift-right: [w556] -> w549
                shift-left: w548 -> [w568]
                stop <- w571 continue-if-true
                n205 = call <vilib>:"Read File+ (string).vi"("count"=0, "line mode (characters:F)"=TRUE, "error in (no error)"=w568, "refnum"=w575) -> ("error out"=w557:errorcluster, "string"=w570:string, "dup refnum"=w569:refnum<file>, "EOF?"=w573:bool)  [unwired: 3 in, 1 out]
                n206 = Unbundle By Name(w557) -> ("status"=w572:bool)
                n207 = Search/Split String(string=w570, search string/char (-)="%" ("search char (-)")) -> (substring before match=w563:string, match + rest of string=w576:string)  [unwired: 1 in, 1 out]
                n208 = Not Or(1:w573, 2:w572) -> (0:w571:bool)
                n209 = String Length(string=w576) -> (length=w562:i32)
                n210 = Subtract(x=w562, y=3) -> (x-y=w565:i32)
                n211 = String Subset(string=w576, offset (0)=1, length (rest)=w565) -> (substring=w560:string)
                n212 = for {
                  N: w558 -> [_]
                  tunnel: w564 -> [w587] mode=indexing
                  tunnel: w563 -> [w582]
                  shift-right: [w583] -> w559
                  shift-left: w561 -> [w584]
                  tunnel: w560 -> [w581]
                  shift-right: [w579] -> w556
                  shift-left: w557 -> [w580]
                  i -> [w585]
                  n213 = Match Pattern(string=w587, regular expression=w582) -> (offset past match=w588:i32)  [unwired: 1 in, 3 out]
                  n214 = Increment(x=w588) -> (x+1=w589:i32)
                  n215 = Greater Than 0?(x=w589) -> (x > 0?=w586:bool)
                  n216 = case shown="True" w586 {
                    tunnel: w585 -> [_ w597]
                    tunnel: w581 -> [_ w596]
                    tunnel: w584 -> [w591 w595]
                    tunnel: [w591 w594] -> w583
                    tunnel: w580 -> [w590 w593]
                    tunnel: [w590 w592] -> w579
                    frame False {
                    }
                    frame True {
                      n217 = case shown="0, Default" w597 {
                        tunnel: w596 -> [w598 w602 w607 w613 w619 w625 w629 w636 w642 w646 w651 w660 w665 w676 w682 w686]
                        tunnel: w595 -> [w600 w604 w608 w615 w621 w627 w632 w633 w639 w647 w652 w663 w668 w678 w681 w689]
                        tunnel: [w601 w605 w609 w614 w620 w626 w631 w634 w640 w648 w653 w662 w667 w677 w679 w687] -> w594
                        tunnel: w593 -> [w599 w603 w606 w610 w616 w622 w630 w635 w641 w649 w654 w655 w664 w675 w680 w688]
                        tunnel: [w599 w603 w606 w610 w616 w622 w630 w635 w641 w649 w654 w655 w664 w675 w680 w688] -> w592
                        frame 0, Default {
                          n218 = Bundle By Name(cluster=w600, "Bias Supply Name"=w598) -> (w601:T5)
                        }
                        frame 1 {
                          n219 = Bundle By Name(cluster=w604, "SMU Name"=w602) -> (w605:T5)
                        }
                        frame 2 {
                          n220 = Bundle By Name(cluster=w608, "LCR Name"=w607) -> (w609:T5)
                        }
                        frame 3 {
                          n221 = Scan Value(string=w613, format string="%.1f") -> (value=w612:dbl)  [unwired: 1 in, 1 out]
                          n222 = Bundle By Name(cluster=w615, "Bias Voltage [V]"=w612) -> (w614:T5)
                        }
                        frame 4 {
                          n223 = Scan Value(string=w619, format string="%.1f") -> (value=w618:dbl)  [unwired: 1 in, 1 out]
                          n224 = Bundle By Name(cluster=w621, "Base Voltage [V]"=w618) -> (w620:T5)
                        }
                        frame 5 {
                          n225 = Scan Value(string=w625, format string="%.1f") -> (value=w624:dbl)  [unwired: 1 in, 1 out]
                          n226 = Bundle By Name(cluster=w627, "Base Ramp Step [V]"=w624) -> (w626:T5)
                        }
                        frame 6 {
                          n227 = Decimal String To Number(string=w629) -> (number=w628:i32)  [unwired: 2 in, 1 out]
                          n228 = Bundle By Name(cluster=w632, "Base Ramp Interval [ms]"=w628) -> (w631:T5)
                        }
                        frame 7 {
                          n229 = Scan Value(string=w636, format string="%.1f") -> (value=w638:dbl)  [unwired: 1 in, 1 out]
                          n230 = Bundle By Name(cluster=w633, "High Voltage [V]"=w638) -> (w634:T5)
                        }
                        frame 8 {
                          n231 = Scan Value(string=w642, format string="%.1f") -> (value=w644:dbl)  [unwired: 1 in, 1 out]
                          n232 = Bundle By Name(cluster=w639, "High Ramp Step [V]"=w644) -> (w640:T5)
                        }
                        frame 9 {
                          n233 = Decimal String To Number(string=w646) -> (number=w645:i32)  [unwired: 2 in, 1 out]
                          n234 = Bundle By Name(cluster=w647, "High Ramp Interval [ms]"=w645) -> (w648:T5)
                        }
                        frame 10 {
                          n235 = Decimal String To Number(string=w651) -> (number=w650:i32)  [unwired: 2 in, 1 out]
                          n236 = Bundle By Name(cluster=w652, "AC frequency [Hz]"=w650) -> (w653:T5)
                        }
                        frame 11 {
                          w659 = u16 0 items=["serial", "parallel"] ("RC Configuration")
                          w658 = u16 1 items=["serial", "parallel"] ("RC Configuration")
                          n237 = Equal?(x=w660, y="serial") -> (x = y?=w657:bool)
                          n238 = Select(t=w659, s=w657, f=w658) -> (s? t:f=w656:u16)
                          n239 = Bundle By Name(cluster=w663, "RC Configuration"=w656) -> (w662:T5)
                        }
                        frame 12 {
                          n240 = Scan Value(string=w665, format string="%.1f") -> (value=w666:dbl)  [unwired: 1 in, 1 out]
                          n241 = Bundle By Name(cluster=w668, "AC amplitude [V]"=w666) -> (w667:T5)
                        }
                        frame 13 {
                          n242 = Equal?(x=w676, y="Arduino") -> (x = y?=w673:bool)
                          n243 = Select(t=enum16{"Read Arduino", "Enter manually"}."Read Arduino" ("Temperature Readout"), s=w673, f=enum16{"Read Arduino", "Enter manually"}."Enter manually" ("Temperature Readout")) -> (s? t:f=w670:enum16{"Read Arduino", "Enter manually"})
                          n244 = Bundle By Name(cluster=w678, "Temperature Readout"=w670) -> (w677:T5)
                        }
                        frame 14 {
                          n245 = Scan Value(string=w682, format string="%.1f") -> (value=w683:dbl)  [unwired: 1 in, 1 out]
                          n246 = Bundle By Name(cluster=w681, "Fraction of good strips [%]"=w683) -> (w679:T5)
                        }
                        frame 15 {
                          n247 = Decimal String To Number(string=w686) -> (number=w685:i32)  [unwired: 2 in, 1 out]
                          n248 = Bundle By Name(cluster=w689, "Probe Card Channels"=w685) -> (w687:T5)
                        }
                      }
                    }
                  }
                }
              }
              n249 = call <vilib>:"Close File+.vi"("error in (no error)"=w549, "refnum"=w550) -> ()  [unwired: 3 in, 3 out]
            }
            frame Error {
              n250 = One Button Dialog(message="Can't open definitions file!") -> ()  [unwired: 1 in, 1 out]
            }
          }
          n251 = global write "QC_MeasurementSetup.vi" "Striptest Measurement Parameters"(w540) -> ()
        }
      }
    }
  }
